vi "FTP.ListFiles.vi"(3 "remote port (21)":u16=21, 5 "password":string="admin", 7 "user":string="admin", 8 "error in (no error)":errorcluster, 10 "directory path":path, 11 "host":string) -> (0 "error out":errorcluster, 2 "directories":string[](array[string]))   [LabVIEW 2016]
uses:
  <vilib>/FTP/ftp2.llb/FTP File Info.ctl
  <vilib>/FTP/NI_FTP.lvlib
panel:
  out "dir list":T1[](array[typedef])
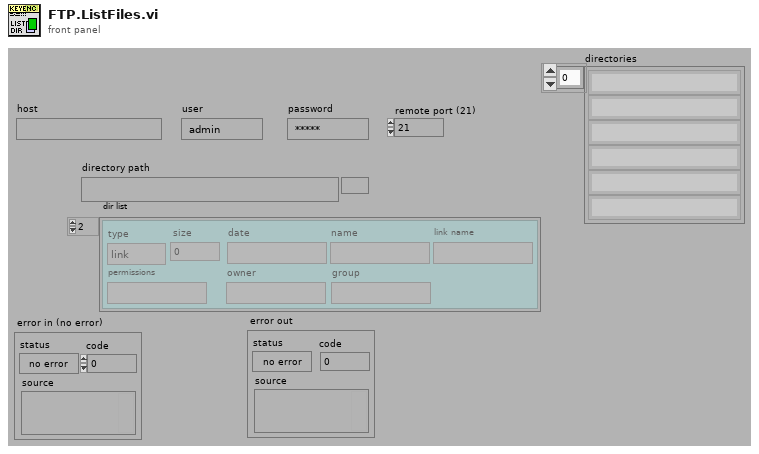
[diagram p1: front panel]
types:
  T1 = typedef "NI_FTP.lvlib/FTP File Info.ctl" = cluster{"type":enum16{"unknown", "file", "dir", "link"}, "permissions":string, "owner":string, "group":string, "size":i32, "date":string, "name":string, "link name":string}
  T2 = typedef "NI_FTP.lvlib/FTP Session.ctl" = refnum<k5>
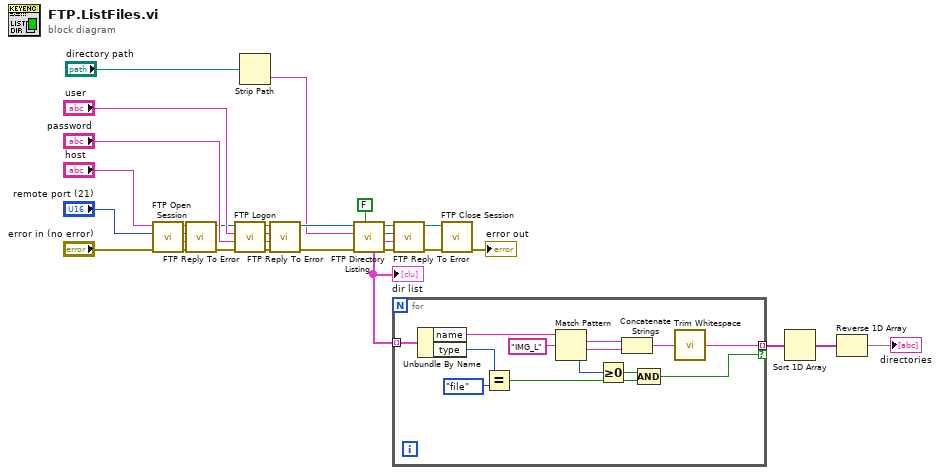
[diagram p0: block diagram]
diagram:
  n1 = call <vilib>:"FTP Open Session.vi"("error in (no error)"="error in (no error)", "remote port (21)"="remote port (21)", "address"="host") -> ("error out"=w27:errorcluster, "reply string"=w24:string, "reply code"=w25:i32, "ftp session"=w26:T2)  [unwired: 5 in]
  n2 = call <vilib>:"FTP Reply To Error.vi"("error in (no error)"=w27, "reply string in"=w24, "reply code in"=w25, "ftp session"=w26) -> ("error out"=w22:errorcluster, "ftp session out"=w23:T2)  [unwired: 2 out]
  n3 = call <vilib>:"FTP Logon.vi"("error in (no error)"=w22, "password"="password", "user"="user", "ftp session"=w23) -> ("error out"=w21:errorcluster, "reply string"=w18:string, "reply code"=w19:i32, "ftp session out"=w20:T2)  [unwired: 4 in]
  n4 = Strip Path(path="directory path") -> (name=w4:string)  [unwired: 1 out]
  n5 = call <vilib>:"FTP Reply To Error.vi"("error in (no error)"=w21, "reply string in"=w18, "reply code in"=w19, "ftp session"=w20) -> ("error out"=w13:errorcluster, "ftp session out"=w7:T2)  [unwired: 2 out]
  n6 = call <vilib>:"FTP Directory Listing.vi"("active (T)"=FALSE, "error in (no error)"=w13, "directory path"=w4, "ftp session"=w7) -> ("error out"=w9:errorcluster, "reply string"=w12:string, "reply code"=w11:i32, "ftp session out"=w10:T2, "dir list"=w6:T1[])  [unwired: 3 in]
  "dir list" <- w6
  n7 = for {
    tunnel: w6 -> [w44] mode=indexing
    tunnel: [w36] -> w2 mode=indexing if=w34
    n8 = Unbundle By Name(w44) -> ("name"=w32:string, "type"=w33:enum16{"unknown", "file", "dir", "link"})
    n9 = Equal?(x=w33, y=enum16{"unknown", "file", "dir", "link"}."file" ("type")) -> (x = y?=w37:bool)
    n10 = Match Pattern(string=w32, regular expression="IMG_L") -> (match substring=w40:string, after substring=w35:string, offset past match=w42:i32)  [unwired: 1 in, 1 out]
    n11 = Greater Or Equal To 0?(x=w42) -> (x >= 0?=w38:bool)
    n12 = Concatenate Strings(w40, w35) -> (w41:string)
    n13 = Compound Arithmetic op=AND(w38, w37) -> (w34:bool)
    n14 = call <vilib>:"Trim Whitespace.vi"("string"=w41) -> ("trimmed string"=w36:string)  [unwired: 1 in]
  }
  n15 = call <vilib>:"FTP Reply To Error.vi"("error in (no error)"=w9, "reply string in"=w12, "reply code in"=w11, "ftp session"=w10) -> ("error out"=w17:errorcluster, "ftp session out"=w16:T2)  [unwired: 2 out]
  n16 = call <vilib>:"FTP Close Session.vi"("error in (no error)"=w17, "ftp session"=w16) -> ("error out"=→"error out":errorcluster)  [unwired: 6 in, 3 out]
  n17 = Sort 1D Array(array=w2) -> (sorted array=w3:string[])
  n18 = Reverse 1D Array(array=w3) -> (reversed array=→"directories":string[])
